vi "Grid SetForcus.vi"(8 "エラー入力（エラーなし）":errorcluster, 10 "EditPos入力":T1 caption="EditPos出力", 11 "Table入力":refnum<vi>) -> (0 "error out":errorcluster caption="エラー出力", 2 "EditPos出力":T1, 3 "Table出力":refnum<vi>)   [LabVIEW 2016]
uses:
  <vilib>/Utility/miscctls.llb/LVRowAndColumnTypeDef.ctl
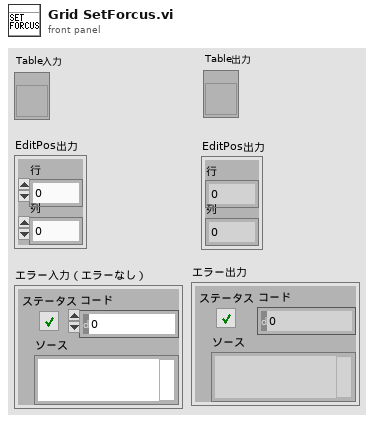
[diagram p1: front panel]
types:
  T1 = typedef "LVRowAndColumnTypeDef.ctl" = cluster{"Row":i32, "Column":i32}
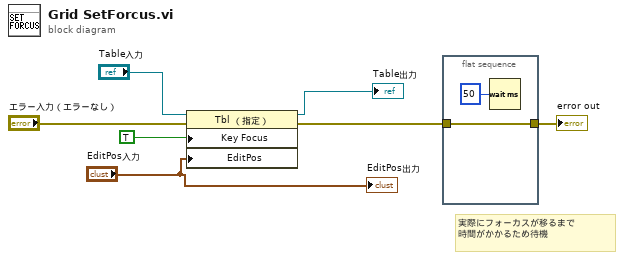
[diagram p0: block diagram]
diagram:
  # "実際にフォーカスが移るまで\n時間がかかるため待機"
  n1 = property on="プロパティノード" class="Tbl （指定）"(reference="Table入力", error in="エラー入力（エラーなし）", "Key Focus"=TRUE, "EditPos"="EditPos入力") -> (reference out=→"Table出力":refnum<vi>, error out=w2:errorcluster)
  n2 = flat-sequence {
    tunnel: w2 -> [w8]
    tunnel: [w8] -> w1
    frame #0 {
      n3 = Wait (ms)(milliseconds to wait=u32 50 ("ミリ秒待機時間")) -> ()  [unwired: 1 out]
    }
  }
  "error out" <- w1
  "EditPos出力" <- "EditPos入力"
